vi "Loop (DMA).vi"(8 "Error IN":errorcluster, 11 "FPGA Ref":T1) -> (0 "Error OUT":errorcluster, 3 "FPGA Ref Out":T1)   [LabVIEW 2013]
uses:
  <vilib>/rvi/interface/nirviMethod/nirviMethod.xnode
  <vilib>/rvi/errors/niLvFpgaMergeErrorWithErrorCode.vi
  Real-Time/Controls/RT FIFO Mode.ctl
  Type Defs/Pump Data Mode.ctl
  <vilib>/FPGAPlugInAG/sbRIO-9626/niLvFpga_ConfigureFifo_sbRIO-9626.vi
  <vilib>/FPGAPlugInAG/sbRIO-9626/niLvFpga_ReadFifo_sbRIO-9626.vi
  Controls/FPGA_Reference.ctl
  FPGA Bitfiles/LSDurability_FPGATarget_LSDurabilityMain_Q3PF1pU0VRY.lvbitx
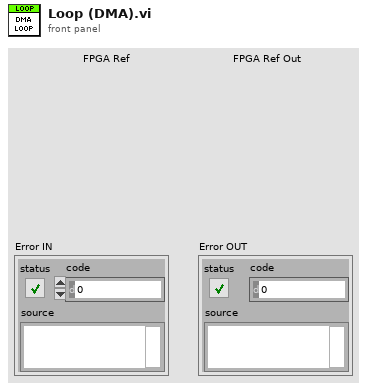
[diagram p1: front panel]
types:
  T1 = typedef "FPGA_Reference.ctl" = refnum<k20>
  T2 = typedef "Pump Data Mode.ctl" = enum16{"Read", "Write Data", "Write Cal", "Write Watlow Data", "Write Pressure Offsets", "Write Initial Times", "Write Pumps Present"}
  T3 = typedef "RT FIFO Mode.ctl" = enum16{"Create", "Write", "Read", "Delete"}
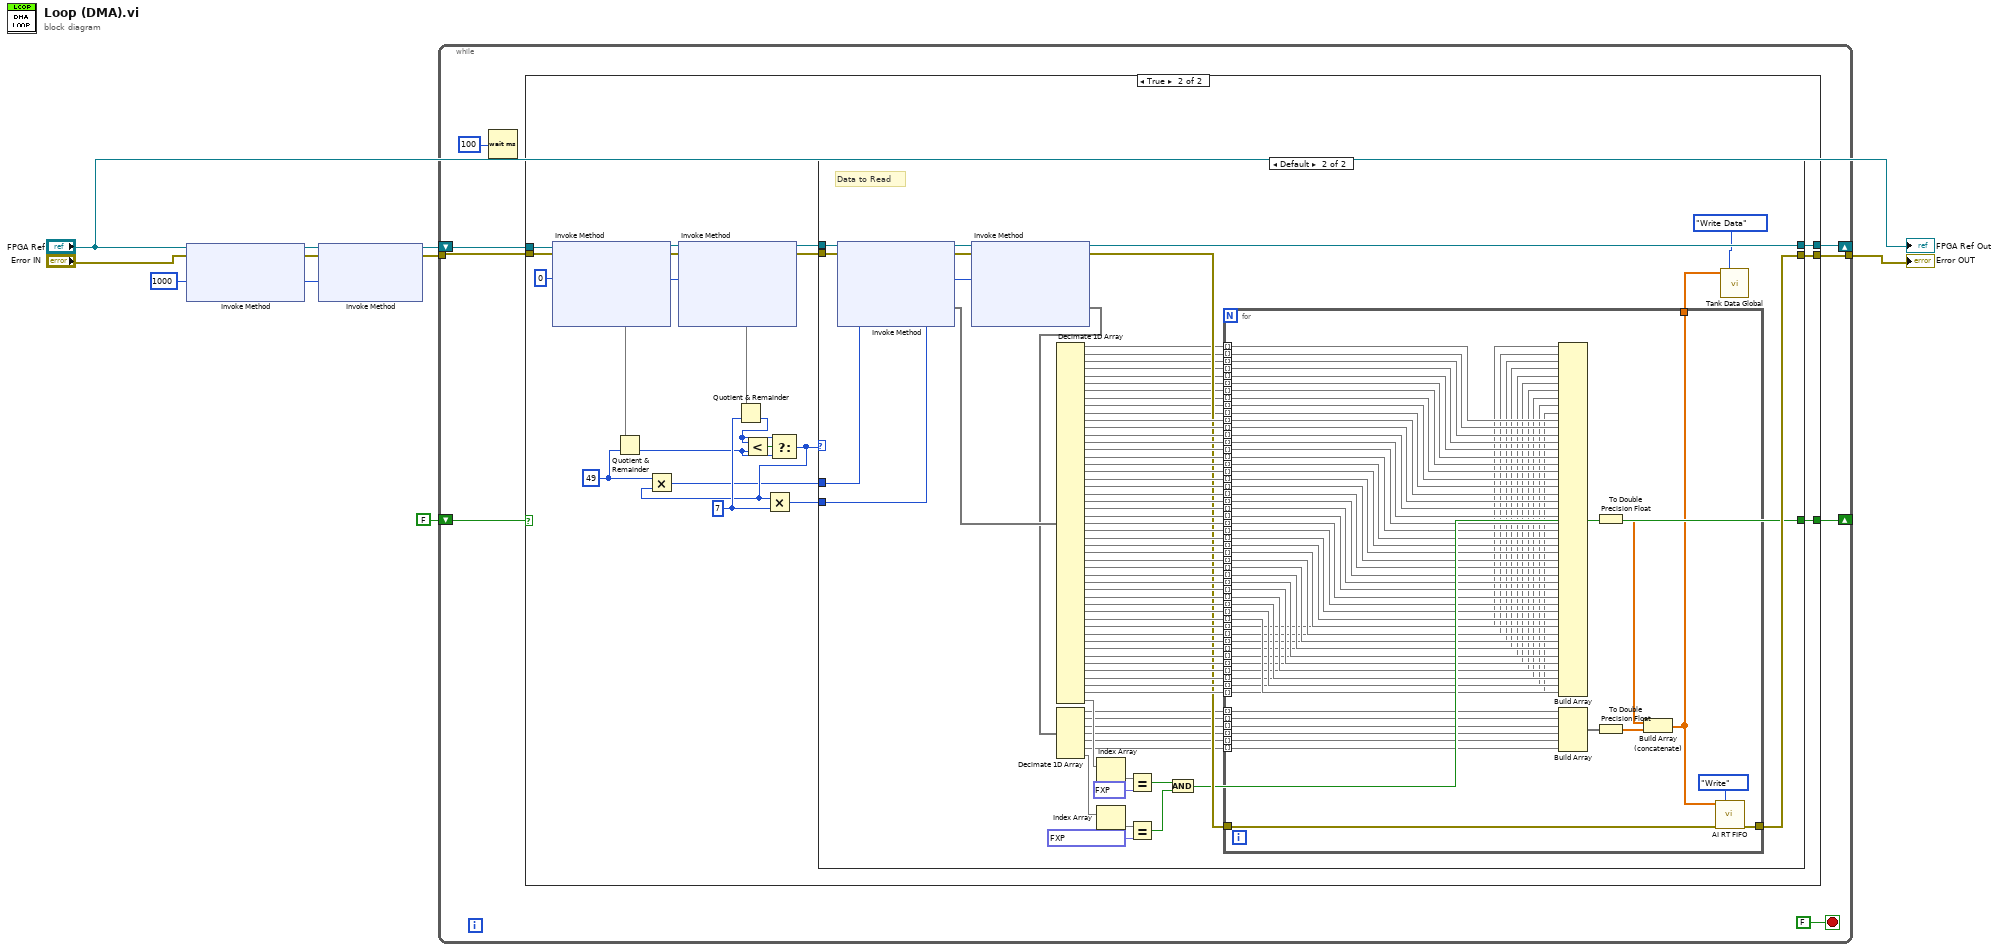
[diagram p0: block diagram]
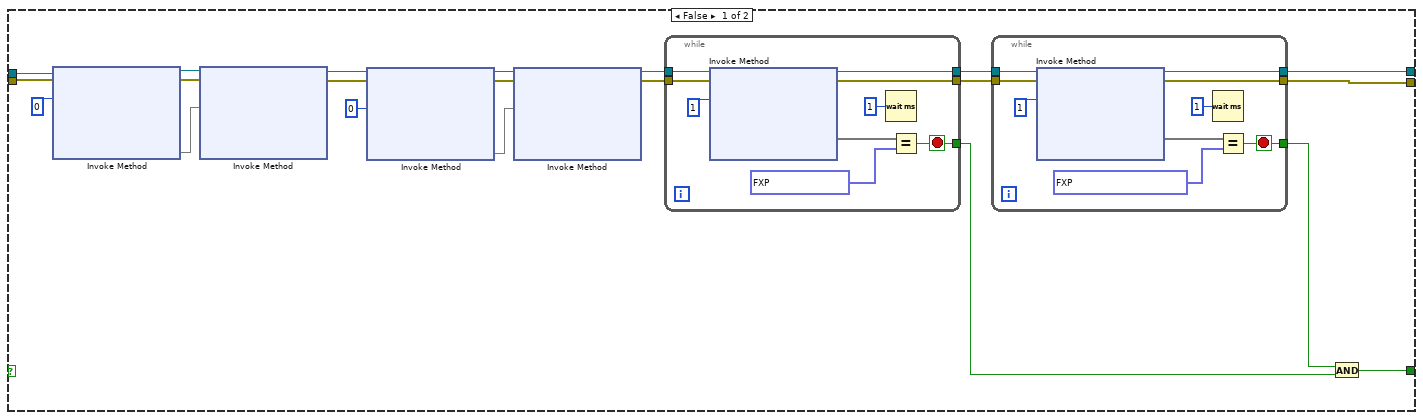
[diagram p2: hidden frame]
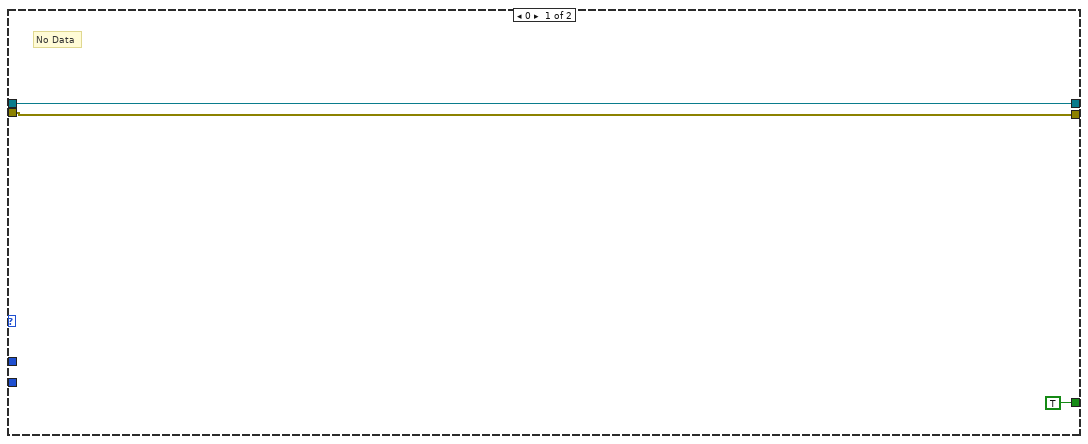
[diagram p3: hidden frame]
diagram:
  w2 = u32 1000 ("Requested Depth")
  n1 = xnode "Invoke Method"("FPGA VI Reference In"="FPGA Ref", "error in"="Error IN", "Requested Depth"=w2) -> ("FPGA VI Reference Out"=w4:T1, "error out"=w3:errorcluster)  [unwired: 1 out]
  n2 = xnode "Invoke Method"("FPGA VI Reference In"=w4, "error in"=w3, "Requested Depth"=w2) -> ("FPGA VI Reference Out"=w7:T1, "error out"=w6:errorcluster)  [unwired: 1 out]
  n3 = while {
    tunnel: w6 -> [w17]
    tunnel: [w16] -> w8
    shift-right: [w15] -> _
    shift-left: FALSE -> [w14]
    shift-right: [w12] -> _
    shift-left: w7 -> [w13]
    stop <- FALSE stop-if-true
    n4 = Wait (ms)(milliseconds to wait=u32 100) -> ()  [unwired: 1 out]
    n5 = case shown="True" w14 {
      tunnel: w17 -> [w38 w76]
      tunnel: [w21 w74] -> w16
      tunnel: [w18 w73] -> w15
      tunnel: w13 -> [w37 w71]
      tunnel: [w22 w72] -> w12
      frame False {
        n6 = xnode "Invoke Method"("FPGA VI Reference In"=w37, "error in"=w38, "Number of Elements"=u32 0) -> ("FPGA VI Reference Out"=w33:T1, "error out"=w35:errorcluster, "Elements Remaining"=w34)  [unwired: 1 in, 1 out]
        n7 = xnode "Invoke Method"("FPGA VI Reference In"=w33, "error in"=w35, "Number of Elements"=w34) -> ("FPGA VI Reference Out"=w30:T1, "error out"=w29:errorcluster)  [unwired: 1 in, 2 out]
        n8 = xnode "Invoke Method"("FPGA VI Reference In"=w30, "error in"=w29, "Number of Elements"=u32 0) -> ("FPGA VI Reference Out"=w28:T1, "error out"=w27:errorcluster, "Elements Remaining"=w32)  [unwired: 1 in, 1 out]
        n9 = xnode "Invoke Method"("FPGA VI Reference In"=w28, "error in"=w27, "Number of Elements"=w32) -> ("FPGA VI Reference Out"=w26:T1, "error out"=w25:errorcluster)  [unwired: 1 in, 2 out]
        n10 = while {
          tunnel: w25 -> [w55]
          tunnel: [w53] -> w23
          tunnel: [w52] -> w19
          tunnel: [w51] -> w24
          tunnel: w26 -> [w50]
          stop <- w52 stop-if-true
          n11 = xnode "Invoke Method"("FPGA VI Reference In"=w50, "error in"=w55, "Number of Elements"=u32 1) -> ("FPGA VI Reference Out"=w51:T1, "error out"=w53:errorcluster, "Data"=w54:void[])  [unwired: 1 in, 1 out]
          n12 = Wait (ms)(milliseconds to wait=u32 1) -> ()  [unwired: 1 out]
          n13 = Equal?(x=w54, y=fxp<+/-,26,15>[] [-9999.0] ("Data")) -> (x = y?=w52:bool)
        }
        n14 = while {
          tunnel: w23 -> [w46]
          tunnel: [w44] -> w21
          tunnel: [w43] -> w20
          tunnel: [w42] -> w22
          tunnel: w24 -> [w41]
          stop <- w43 stop-if-true
          n15 = xnode "Invoke Method"("FPGA VI Reference In"=w41, "error in"=w46, "Number of Elements"=u32 1) -> ("FPGA VI Reference Out"=w42:T1, "error out"=w44:errorcluster, "Data"=w45:void[])  [unwired: 1 in, 1 out]
          n16 = Wait (ms)(milliseconds to wait=u32 1) -> ()  [unwired: 1 out]
          n17 = Equal?(x=w45, y=fxp<+,40,40>[] [1099511627775.0] ("Data")) -> (x = y?=w43:bool)
        }
        n18 = And(x=w20, y=w19) -> (x .and. y?=w18:bool)
      }
      frame True {
        w60 = u32 49 ("y")
        w70 = u32 7 ("y")
        w65 = u32 0 ("Number of Elements")
        n19 = xnode "Invoke Method"("FPGA VI Reference In"=w71, "error in"=w76, "Number of Elements"=w65) -> ("FPGA VI Reference Out"=w69:T1, "error out"=w68:errorcluster, "Elements Remaining"=w75)  [unwired: 1 in, 1 out]
        n20 = Quotient & Remainder(x=w75, y=w60) -> (floor(x/y)=w62:u32)  [unwired: 1 out]
        n21 = xnode "Invoke Method"("FPGA VI Reference In"=w69, "error in"=w68, "Number of Elements"=w65) -> ("FPGA VI Reference Out"=w67:T1, "error out"=w66:errorcluster, "Elements Remaining"=w64)  [unwired: 1 in, 1 out]
        n22 = Quotient & Remainder(x=w64, y=w70) -> (floor(x/y)=w61:u32)  [unwired: 1 out]
        n23 = Less?(x=w61, y=w62) -> (x < y?=w63:bool)
        n24 = Select(t=w61, s=w63, f=w62) -> (s? t:f=w59:u32)
        n25 = Multiply(x=w60, y=w59) -> (x*y=w58:u32)
        n26 = Multiply(x=w59, y=w70) -> (x*y=w57:u32)
        n27 = case shown="Default" w59 {
          tunnel: [w77 w111] -> w72
          tunnel: w66 -> [w79 w155]
          tunnel: [w79 w152] -> w74
          tunnel: [TRUE w91] -> w73
          tunnel: w67 -> [w77 w153]
          tunnel: w58 -> [_ w110]
          tunnel: w57 -> [_ w109]
          frame 0 {
            # "No Data"
          }
          frame Default {
            # "Data to Read"
            n28 = xnode "Invoke Method"("FPGA VI Reference In"=w153, "error in"=w155, "Number of Elements"=w110) -> ("FPGA VI Reference Out"=w112:T1, "error out"=w108:errorcluster, "Data"=w140:void[])  [unwired: 1 in, 1 out]
            n29 = xnode "Invoke Method"("FPGA VI Reference In"=w112, "error in"=w108, "Number of Elements"=w109) -> ("FPGA VI Reference Out"=w111:T1, "error out"=w107:errorcluster, "Data"=w105:void[])  [unwired: 1 in, 1 out]
            n30 = Decimate 1D Array(w140) -> (w80:void[], w81:void[], w82:void[], w83:void[], w84:void[], w85:void[], w86:void[], w87:void[], w88:void[], w89:void[], w151:void[], w150:void[], w149:void[], w148:void[], w147:void[], w146:void[], w145:void[], w144:void[], w143:void[], w142:void[], w141:void[], w139:void[], w138:void[], w137:void[], w136:void[], w135:void[], w134:void[], w133:void[], w132:void[], w131:void[], w130:void[], w129:void[], w128:void[], w127:void[], w126:void[], w125:void[], w124:void[], w123:void[], w122:void[], w121:void[], w120:void[], w119:void[], w118:void[], w117:void[], w116:void[], w115:void[], w114:void[], w113:void[], w106:void[])
            n31 = Decimate 1D Array(w105) -> (w104:void[], w103:void[], w102:void[], w101:void[], w100:void[], w99:void[], w97:void[])
            n32 = Index Array(array=w106) -> (element=w154)  [unwired: 1 in]
            n33 = Index Array(array=w97) -> (element=w96)  [unwired: 1 in]
            n34 = Equal?(x=w154, y=fxp<+/-,26,15> -9999.0) -> (x = y?=w92:bool)
            n35 = Equal?(x=w96, y=fxp<+,40,40> 1099511627775.0) -> (x = y?=w93:bool)
            n36 = And(x=w92, y=w93) -> (x .and. y?=w91:bool)
            n37 = for {
              tunnel: w107 -> [w216]
              tunnel: [w215] -> w152
              tunnel: w151 -> [w211] mode=indexing
              tunnel: w150 -> [w210] mode=indexing
              tunnel: w149 -> [w209] mode=indexing
              tunnel: w148 -> [w214] mode=indexing
              tunnel: w147 -> [w213] mode=indexing
              tunnel: w146 -> [w212] mode=indexing
              tunnel: w145 -> [w208] mode=indexing
              tunnel: w144 -> [w207] mode=indexing
              tunnel: w143 -> [w206] mode=indexing
              tunnel: w142 -> [w188] mode=indexing
              tunnel: w141 -> [w205] mode=indexing
              tunnel: w139 -> [w204] mode=indexing
              tunnel: w138 -> [w203] mode=indexing
              tunnel: w137 -> [w202] mode=indexing
              tunnel: w136 -> [w201] mode=indexing
              tunnel: w135 -> [w200] mode=indexing
              tunnel: w134 -> [w199] mode=indexing
              tunnel: w133 -> [w198] mode=indexing
              tunnel: w132 -> [w197] mode=indexing
              tunnel: w131 -> [w187] mode=indexing
              tunnel: w130 -> [w196] mode=indexing
              tunnel: w129 -> [w195] mode=indexing
              tunnel: [w176] -> w98
              tunnel: w128 -> [w194] mode=indexing
              tunnel: w127 -> [w193] mode=indexing
              tunnel: w126 -> [w192] mode=indexing
              tunnel: w125 -> [w191] mode=indexing
              tunnel: w124 -> [w190] mode=indexing
              tunnel: w123 -> [w189] mode=indexing
              tunnel: w122 -> [w165] mode=indexing
              tunnel: w121 -> [w164] mode=indexing
              tunnel: w120 -> [w163] mode=indexing
              tunnel: w119 -> [w162] mode=indexing
              tunnel: w118 -> [w161] mode=indexing
              tunnel: w117 -> [w160] mode=indexing
              tunnel: w116 -> [w159] mode=indexing
              tunnel: w115 -> [w158] mode=indexing
              tunnel: w114 -> [w157] mode=indexing
              tunnel: w113 -> [w156] mode=indexing
              tunnel: w104 -> [w186] mode=indexing
              tunnel: w103 -> [w185] mode=indexing
              tunnel: w102 -> [w184] mode=indexing
              tunnel: w101 -> [w183] mode=indexing
              tunnel: w100 -> [w182] mode=indexing
              tunnel: w99 -> [w181] mode=indexing
              tunnel: w89 -> [w175] mode=indexing
              tunnel: w88 -> [w174] mode=indexing
              tunnel: w87 -> [w173] mode=indexing
              tunnel: w86 -> [w172] mode=indexing
              tunnel: w85 -> [w171] mode=indexing
              tunnel: w84 -> [w170] mode=indexing
              tunnel: w83 -> [w169] mode=indexing
              tunnel: w82 -> [w168] mode=indexing
              tunnel: w81 -> [w167] mode=indexing
              tunnel: w80 -> [w166] mode=indexing
              n38 = Build Array(w165, w164, w163, w162, w161, w160, w159, w158, w157, w156, w166, w167, w168, w169, w170, w171, w172, w173, w174, w175, w211, w210, w209, w214, w213, w212, w208, w207, w206, w188, w205, w204, w203, w202, w201, w200, w199, w198, w197, w187, w196, w195, w194, w193, w192, w191, w190, w189) -> (w180:void[])
              n39 = Build Array(w186, w185, w184, w183, w182, w181) -> (w179:void[])
              n40 = To Double Precision Float(number=w180) -> (double precision float=w178:dbl[])
              n41 = To Double Precision Float(number=w179) -> (double precision float=w177:dbl[])
              n42 = Build Array (concatenate)(w178, w177) -> (w176:dbl[])
              n43 = call "AI RT FIFO.vi"("Data IN"=w176, "Mode"=RT_FIFO_Mode."Write", "Error IN"=w216) -> ("Error OUT"=w215:errorcluster)  [unwired: 10 in, 2 out]
            }
            n44 = call "Tank Data Global.vi"("Tank Data IN"=w98, "Pump Data Mode"=Pump_Data_Mode."Write Data") -> ()  [unwired: 10 in, 4 out]
          }
        }
      }
    }
  }
  "Error OUT" <- w8
  "FPGA Ref Out" <- "FPGA Ref"
